vi "To Variant.vi"(8 "error in":errorcluster, 11 "Boolean in":refnum<class "Boolean 1D.lvclass">) -> (0 "error out":errorcluster, 3 "Variant":variant)   [LabVIEW 2017, in "Boolean 1D.lvclass"]
uses:
  <vilib>/gpm_packages/@cs/data-type-serializer/source/Boolean 1D/Boolean 1D.lvclass
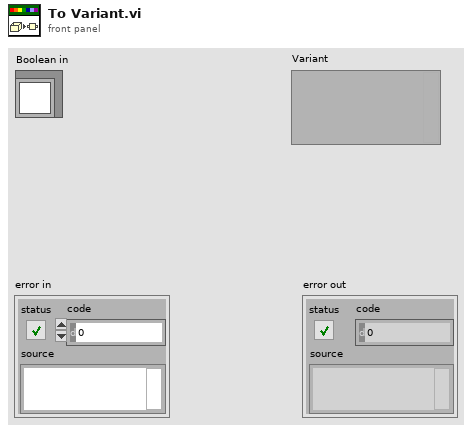
[diagram p1: front panel]
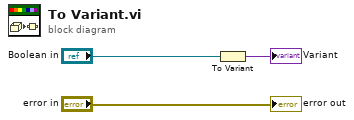
[diagram p0: block diagram]
diagram:
  n1 = To Variant(anything="Boolean in") -> (Variant=→"Variant":variant)
  "error out" <- "error in"
